vi "Add Channel.vi"(7 "highlight (F)":bool, 8 "error in":errorcluster, 9 "channel definition":T2, 10 "name":string, 11 "frame ref in":T1 format="%.0x") -> (0 "error out":errorcluster, 2 "channel ref out":T1 format="%.0x", 3 "frame ref out":T1 format="%.0x")   [LabVIEW 2020, in "AIM ARINC 664 Scripting.lvlib"]
uses:
  AIM ARINC 664 Scripting.lvlib
  <vilib>/NI VeriStand/Custom Device API/Custom Device Item Ref.ctl
  <vilib>/NI VeriStand/Custom Device API/Custom Device Channel.ctl
  <vilib>/NI VeriStand/Custom Device API/Custom Device Channel Type.ctl
  Constants.vi
  <vilib>/NI VeriStand/Custom Device API/Custom Device API.lvlib
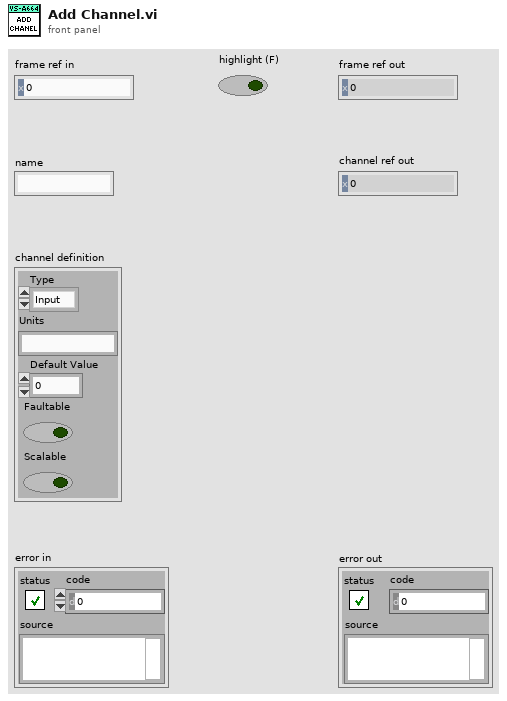
[diagram p1: front panel]
types:
  T1 = typedef "Custom Device API.lvlib/Custom Device Item Ref.ctl" = u64
  T2 = typedef "Custom Device API.lvlib/Custom Device Channel.ctl" = cluster{"Type":T3, "Units":string, "Default Value":dbl, "Faultable":bool, "Scalable":bool}
  T3 = typedef "Custom Device API.lvlib/Custom Device Channel Type.ctl" = enum16{"Input", "Output"}
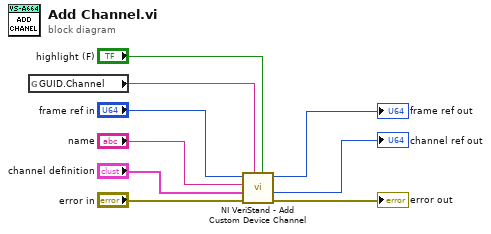
[diagram p0: block diagram]
diagram:
  n1 = global read "Constants.vi" "GUID.Channel"() -> (w1:string)
  n2 = call <vilib>:"NI VeriStand - Add Custom Device Channel.vi"("Highlight? (F)"="highlight (F)", "GUID (Default Channel)"=w1, "error in (no error)"="error in", "Channel"="channel definition", "Channel Name"="name", "Parent Ref in"="frame ref in") -> ("error out"=→"error out":errorcluster, "Channel Ref"=→"channel ref out":T1, "Parent Ref out"=→"frame ref out":T1)  [unwired: 2 in, 1 out]
